vi "Save Sequence Data v1.00.vi"(4 "Parameters":T1={"Magnetic Field"=0.0, "Temperature"=0.0, "Exposure Time"=0.0, "Mag ID string"="", "User Name"="", "Comments"="", "SaveComments?"=1, "X-Axis Unit"=1, "Delimitor"=0, "File Format"=0, "Sample Name"="Sample1"} {"File Format" items=["Macintosh (EOL: CR)", "Unix (EOL: LF)", "DOS/Windows (EOL: CR+LF)"]; "Delimitor" items=["TAB", "COMMA", "SPACE"]; "X-Axis Unit" items=["Point #", "nm", "eV", "meV", "cm-1"]; "SaveComments?" items=["Bare data only", "Saved in the Header Area", "Saved as a Parameter File"]; "Exposure Time" format="%.2f"; "Temperature" format="%.2f"; "Magnetic Field" format="%.2f"}, 5 "Iteration":i32, 7 "File Name":string, 8 "Directory Path":path=path "/DATA") -> (0 "Contents Written":string, 2 "Output File Name":string, 3 "Final File path":path)   [LabVIEW 2020]
uses:
  Globals and TypeDefs/Global Varibal Control.vi
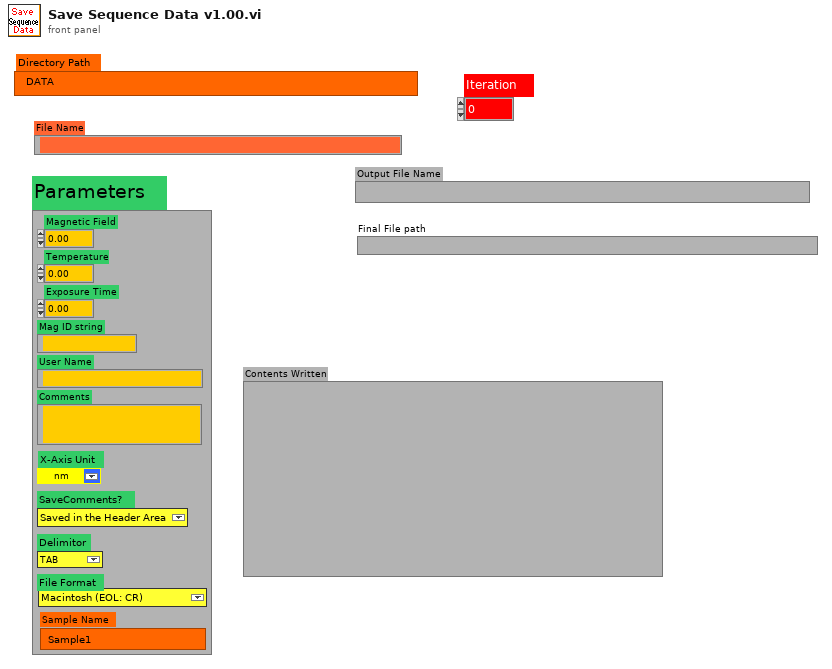
[diagram p1: front panel]
types:
  T1 = cluster{"Magnetic Field":dbl, "Temperature":dbl, "Exposure Time":dbl, "Mag ID string":string, "User Name":string, "Comments":string, "SaveComments?":u16, "X-Axis Unit":u16, "Delimitor":u16, "File Format":u16, "Sample Name":string}
  T2 = enum16{"open", "open or create", "create or replace", "create"}
  T3 = enum32{"existing file", "new file", "new or existing file", "existing dir", "new dir", "new or existing dir", "existing file (use LLBs)", "new file (use LLBs)", "new or existing file (use LLBs)", "new or existing file or directory (use LLBs)", "existing dir (use LLBs)", "new dir (use LLBs)", "new or existing dir (use LLBs)", "existing file or dir", "new file or dir", "new or existing file or dir", "existing file or dir (use LLBs)", "new file or dir (use LLBs)"}
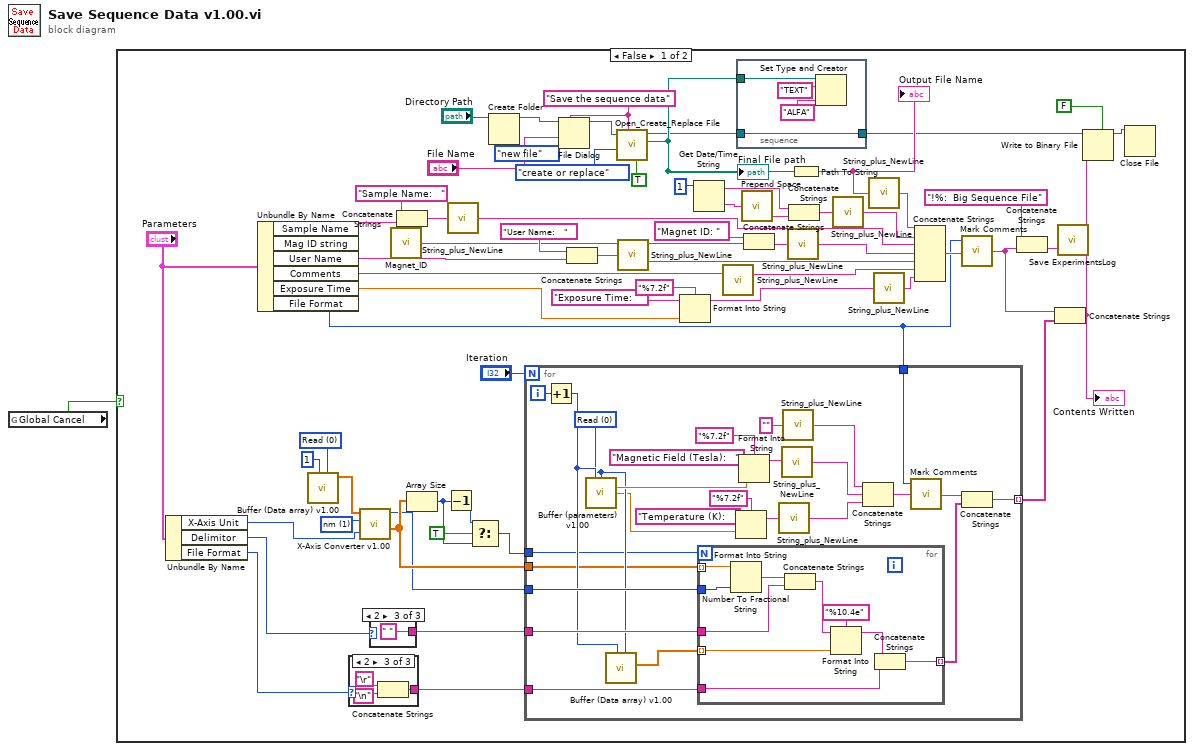
[diagram p0: block diagram]
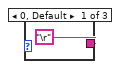
[diagram p2: hidden frame]
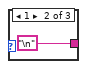
[diagram p3: hidden frame]
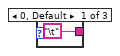
[diagram p4: hidden frame]
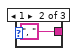
[diagram p5: hidden frame]
diagram:
  n1 = global read "Global Varibal Control.vi" "Global Cancel"() -> (w1:bool)
  n2 = case shown="False" w1 {
    frame False {
      w11 = 1 items=["Point #", "nm", "eV", "meV", "cm-1"] ("Old X-Axis Unit")
      w13 = u16 0 items=["Read", "Write", "Initialize"] ("Read(0) or Write(1)")
      (unwired) T3."new file" ("select mode (2)")
      w42 = "Save the sequence data" ("prompt")
      n3 = Unbundle By Name("Parameters") -> ("X-Axis Unit"=w10:u16, "Delimitor"=w31:u16, "File Format"=w30:u16)
      n4 = Unbundle By Name("Parameters") -> ("Sample Name"=w20:string, "User Name"=w40:string, "Comments"=w25:string, "Exposure Time"=w35:dbl, "File Format"=w28:u16)  [unwired: 1 out]
      n5 = call "Buffer (Data array) v1.00.vi"("Action"=w13, "Read#"=1 ("Buffer Size or Read#")) -> ("X-Data out"=w12:dbl[])  [unwired: 6 in, 3 out]
      n6 = case shown="2" w30 {
        tunnel: ["\r" "\n" w67] -> w32
        frame 0, Default {
        }
        frame 1 {
        }
        frame 2 {
          n7 = Concatenate Strings("\r", "\n") -> (w67:string)
        }
      }
      n8 = call "X-Axis Converter v1.00.vi"("X-Axis Unit"=w10, "Old X-Axis Unit"=w11, "X-Axis input"=w12) -> ("X-Axis Output"=w9:dbl[], "Precision"=w4:i32)  [unwired: 2 in, 2 out]
      n9 = case shown="2" w31 {
        tunnel: ["\t" ", " " "] -> w33
        frame 0, Default {
        }
        frame 1 {
        }
        frame 2 {
        }
      }
      n10 = call "Magnet_ID.vi"() -> ("Cell"=w3:string)
      n11 = Concatenate Strings("Sample Name:   ", w20) -> (w19:string)
      n12 = Array Size(array=w9) -> (size(s)=w6:i32)
      n13 = Decrement(x=w6) -> (x-1=w7:i32)
      n14 = call "String_plus_NewLine.vi"("Input String"=w19) -> ("Input String +[\\n]"=w18:string)
      n15 = Select(t=w7, s=TRUE, f=w6) -> (s? t:f=w5:i32)
      n16 = Create Folder(path (use dialog)="Directory Path") -> (created path=w44:path)  [unwired: 2 in, 2 out]
      n17 = for {
        N: "Iteration" -> [_]
        tunnel: w33 -> [w86]
        tunnel: w32 -> [w85]
        tunnel: w4 -> [w84]
        tunnel: w28 -> [w82]
        tunnel: [w79] -> w27 mode=indexing
        tunnel: w9 -> [w74]
        tunnel: w5 -> [w73]
        i -> [w98]
        w76 = u16 0 items=["Read", "Write", "Initialize"] ("Read(0) or Write(1)")
        n18 = Increment(x=w98) -> (x+1=w77:i32)
        n19 = call "Buffer (parameters) v1.00.vi"("Read#"=w77, "Action"=w76) -> ("Field Out"=w94:dbl, "Temperature Out"=w75:dbl)  [unwired: 9 in, 3 out]
        n20 = call "Buffer (Data array) v1.00.vi"("Action"=w76, "Read#"=w77) -> ("Y-Data out"=w78:dbl[])  [unwired: 6 in, 3 out]
        n21 = for {
          N: w73 -> [_]
          tunnel: w78 -> [w103] mode=indexing
          tunnel: w74 -> [w106] mode=indexing
          tunnel: w84 -> [w107]
          tunnel: w86 -> [w105]
          tunnel: w85 -> [w100]
          tunnel: [w99] -> w80 mode=indexing
          n22 = Number To Fractional String(number=w106, precision (6)=w107) -> (F-format string=w108:string)  [unwired: 2 in]
          n23 = Concatenate Strings(w108, w105) -> (w104:string)
          n24 = Format Into String(format string="%10.4e", initial string=w104, w103) -> (resulting string=w101:string)  [unwired: 1 in, 1 out]
          n25 = Concatenate Strings(w101, w100) -> (w99:string)
        }
        n26 = Format Into String(format string="%7.2f", initial string="Temperature (K):   ", w75) -> (resulting string=w93:string)  [unwired: 1 in, 1 out]
        n27 = Format Into String(format string="%7.2f", initial string="Magnetic Field (Tesla):   ", w94) -> (resulting string=w96:string)  [unwired: 1 in, 1 out]
        n28 = call "String_plus_NewLine.vi"("Input String"=w93) -> ("Input String +[\\n]"=w89:string)
        n29 = call "String_plus_NewLine.vi"("Input String"=w96) -> ("Input String +[\\n]"=w90:string)
        n30 = call "String_plus_NewLine.vi"("Input String"="") -> ("Input String +[\\n]"=w87:string)
        n31 = Concatenate Strings(w87, w90, w89) -> (w83:string)
        n32 = call "Mark Comments.vi"("Input String"=w83, "File Format"=w82) -> ("Output String"=w81:string)  [unwired: 1 in]
        n33 = Concatenate Strings(w81, w80) -> (w79:string)
      }
      n34 = File Dialog(7:w42, 9:"File Name", 11:w44) -> (3:w43:path)  [unwired: 4 in, 3 out]
      n35 = Concatenate Strings("User Name:   ", w40) -> (w53:string)
      n36 = call <vilib>:"Open_Create_Replace File.vi"("advisory dialog? (display:T)"=TRUE, "prompt"=w42, "function (open:0)"=T2."create or replace", "file path"=w43) -> ("new file path"=w24:path, "refnum"=w23:refnum<file>)  [unwired: 4 in, 2 out]
      "Final File path" <- w24
      n37 = call "String_plus_NewLine.vi"("Input String"=w53) -> ("Input String +[\\n]"=w52:string)
      n38 = Format Into String(format string="%7.2f", initial string="Exposure Time:   ", w35) -> (resulting string=w36:string)  [unwired: 1 in, 1 out]
      n39 = Get Date/Time String(date format (0)=1) -> (date string=w61:string, time string=w63:string)  [unwired: 2 in]
      n40 = call "String_plus_NewLine.vi"("Input String"=w25) -> ("Input String +[\\n]"=w26:string)
      n41 = stacked-sequence {
        tunnel: w24 -> [w110]
        tunnel: [w109] -> w22
        tunnel: w23 -> [w109]
        frame #0 {
          n42 = Set Type and Creator(5:"ALFA", 6:"TEXT", 7:w110) -> ()  [unwired: 1 in, 2 out]
        }
      }
      n43 = call "Prepend Space.vi"("Input String"=w63) -> ("Space + Input String"=w62:string)
      n44 = Concatenate Strings("Magnet ID: ", w3) -> (w56:string)
      n45 = call "String_plus_NewLine.vi"("Input String"=w56) -> ("Input String +[\\n]"=w55:string)
      n46 = Concatenate Strings(w61, w62) -> (w60:string)
      n47 = Path To String(path=w24) -> (string=w46:string)
      "Output File Name" <- w46
      n48 = call "String_plus_NewLine.vi"("Input String"=w60) -> ("Input String +[\\n]"=w59:string)
      n49 = call "String_plus_NewLine.vi"("Input String"=w46) -> ("Input String +[\\n]"=w58:string)
      n50 = call "String_plus_NewLine.vi"("Input String"=w36) -> ("Input String +[\\n]"=w39:string)
      n51 = Concatenate Strings(w58, w59, w18, w55, w52, w26, w39) -> (w29:string)
      n52 = call "Mark Comments.vi"("Input String"=w29, "File Format"=w28) -> ("Output String"=w17:string)  [unwired: 1 in]
      n53 = Concatenate Strings("!%:  Big Sequence File", w17) -> (w15:string)
      n54 = Concatenate Strings(w17, w27) -> (w50:string)
      "Contents Written" <- w50
      n55 = call "Save ExperimentsLog.vi"("Contents Written"=w15) -> ()  [unwired: 2 in]
      n56 = Write to Binary File(file (use dialog)=w22, data=w50, 5:FALSE ("prepend array or string size? (T)")) -> (refnum out=w49:refnum<file>)  [unwired: 3 in, 2 out]
      n57 = Close File(refnum=w49) -> ()  [unwired: 1 in, 2 out]
    }
    frame True {
    }
  }
